vi "1WIRE_ROM_SEARCH.vi"(7 "1-Wire DIO Pin":refnum<k21>="ConnectorA/DIO15", 8 "Error In":errorcluster) -> (0 "Error Out":errorcluster, 2 "ROM Array":u64[](array[numeric]))   [LabVIEW 2014]
uses:
  <vilib>/rvi/Emulation/niFpgaGetClockAttributes.vi
  <vilib>/rvi/Emulation/niFpgaSctlEmulationGetInTimedLoop.vi
  <vilib>/rvi/Emulation/niFpgaEmulationReportErrorSimple.vi
  <vilib>/rvi/Emulation/niFpgaCriticalErrorInLSC.vi
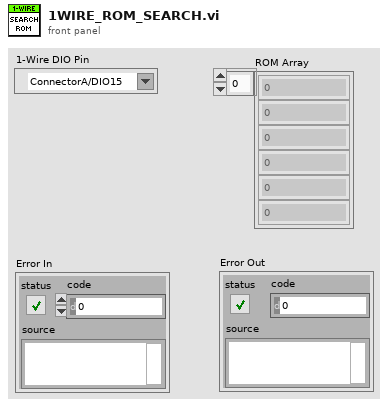
[diagram p1: front panel]
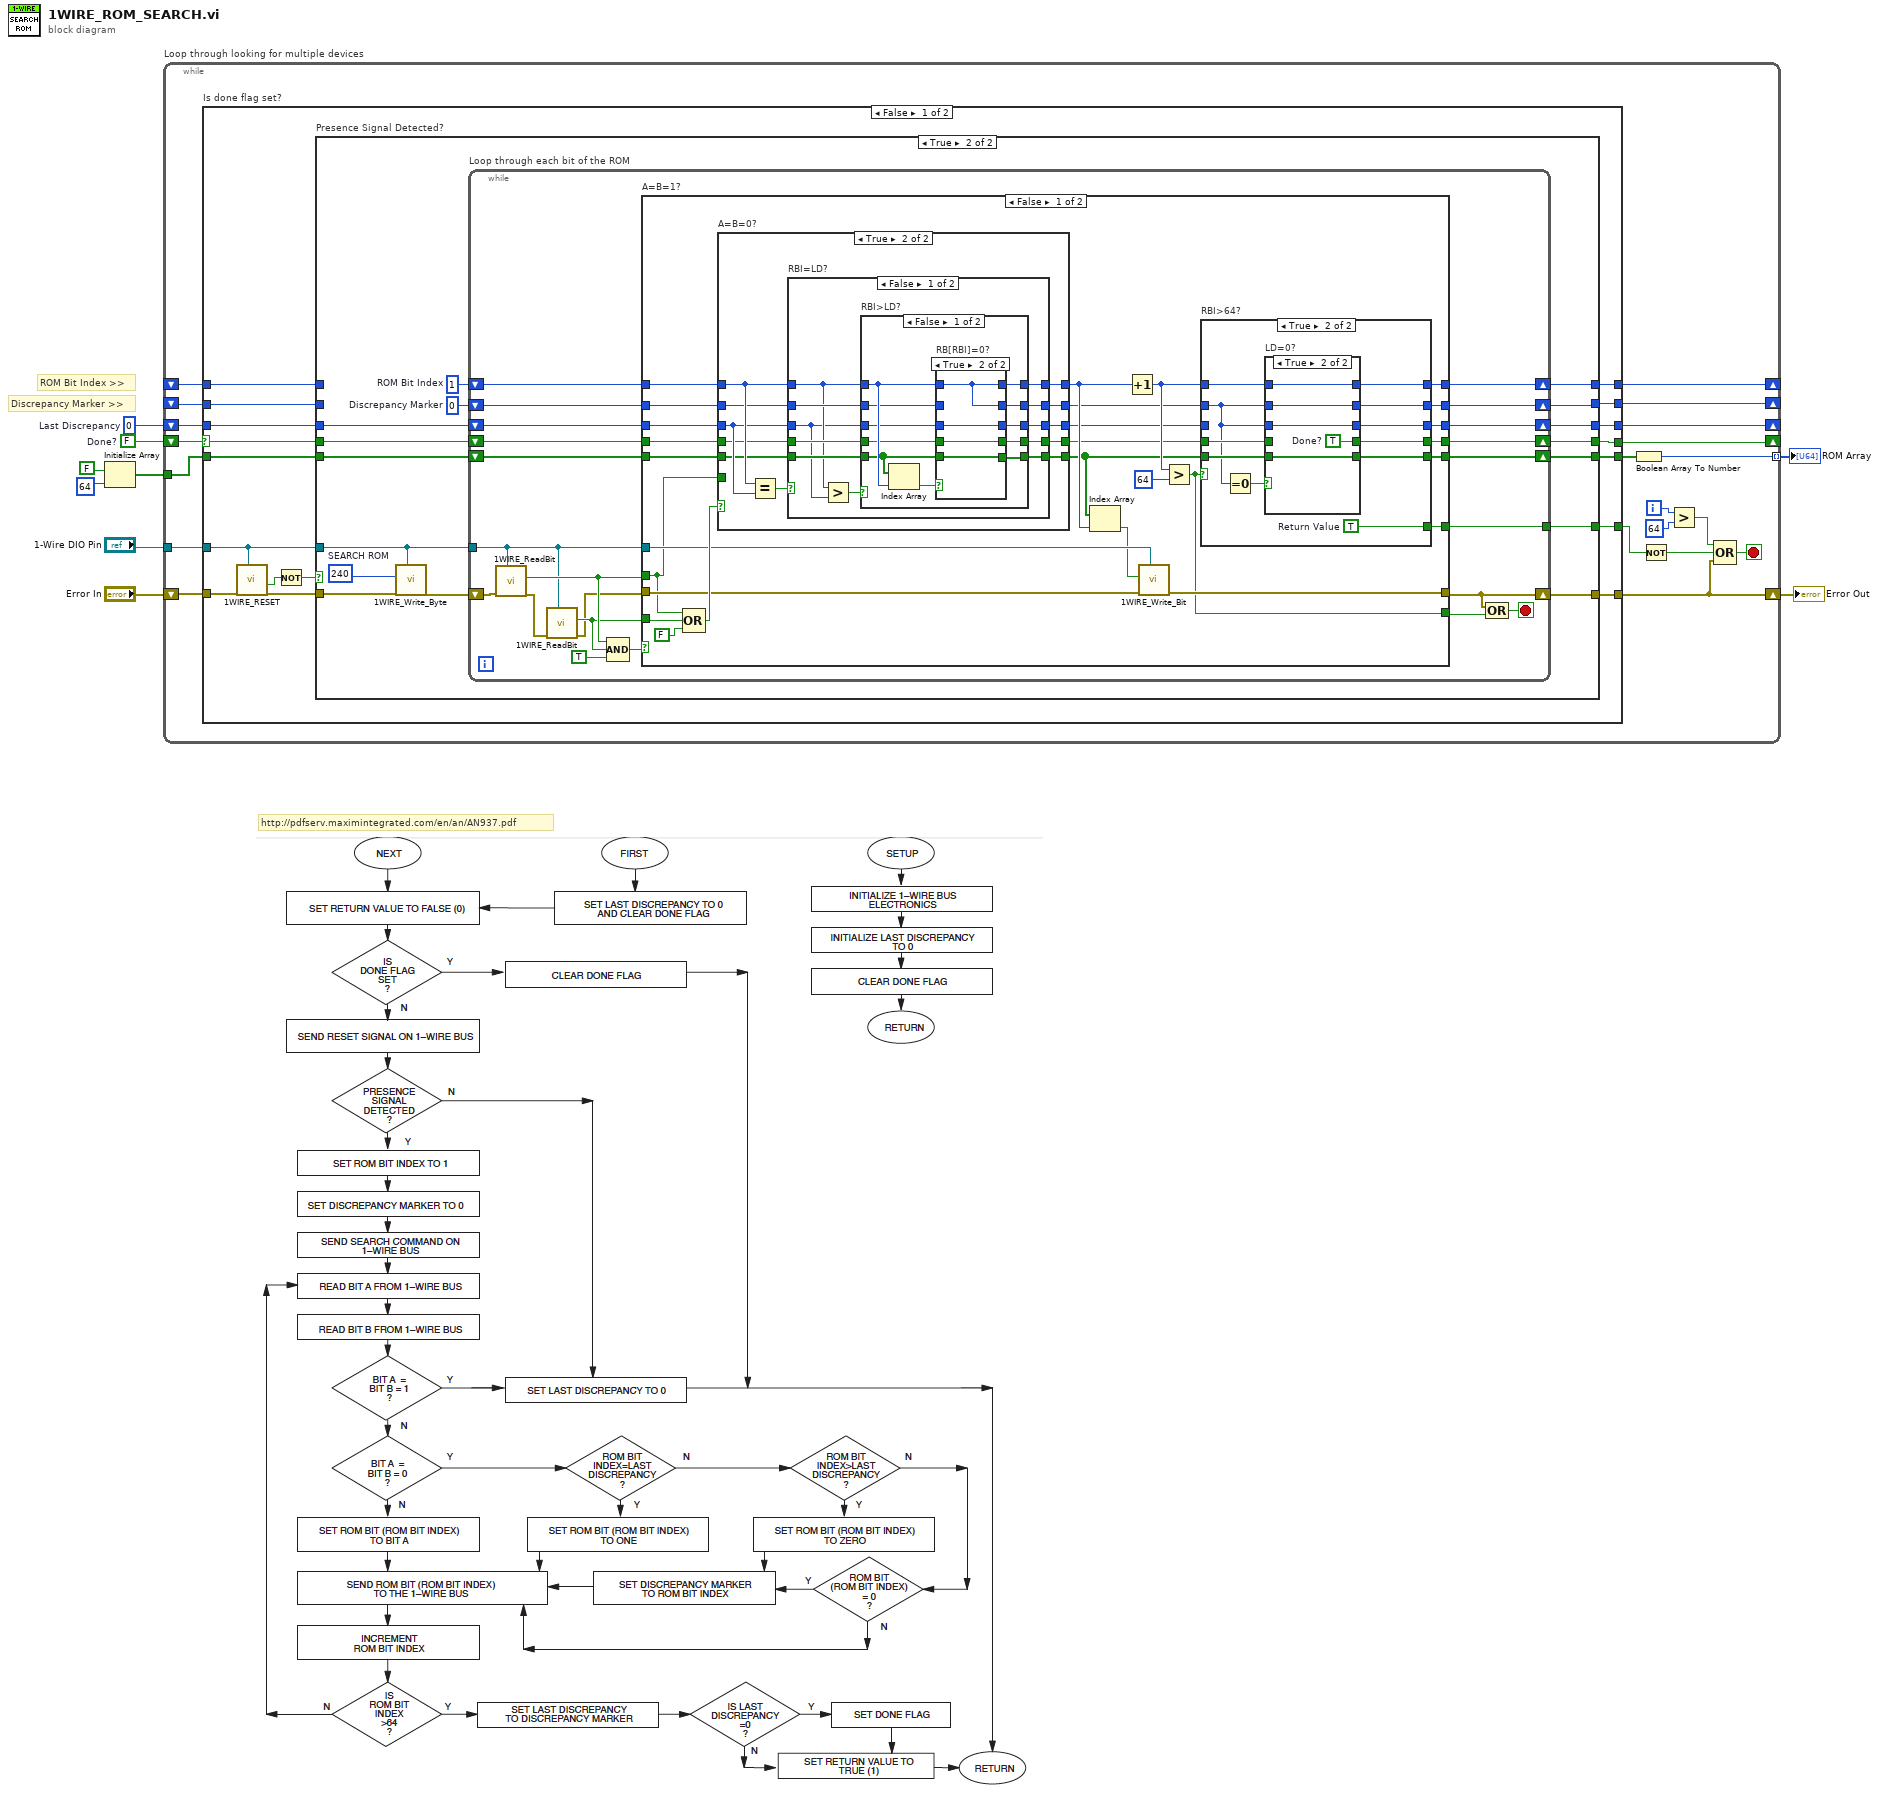
[diagram p0: block diagram]
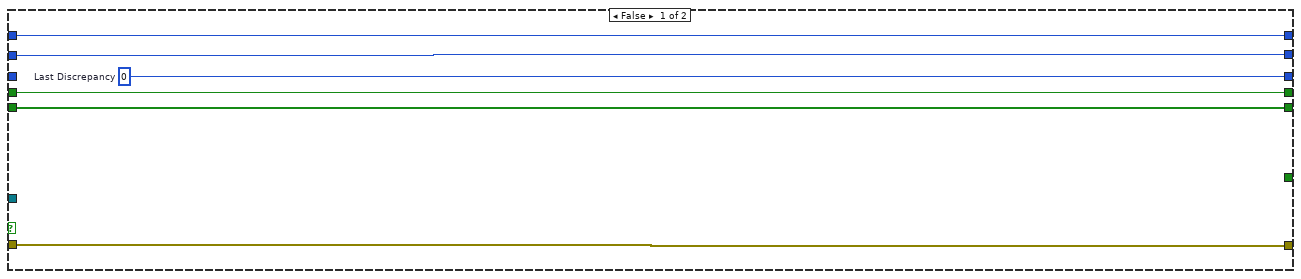
[diagram p2: hidden frame]
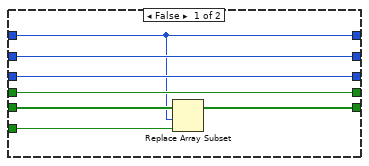
[diagram p5: hidden frame]
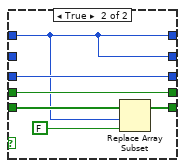
[diagram p7: hidden frame]
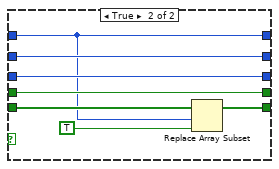
[diagram p8: hidden frame]
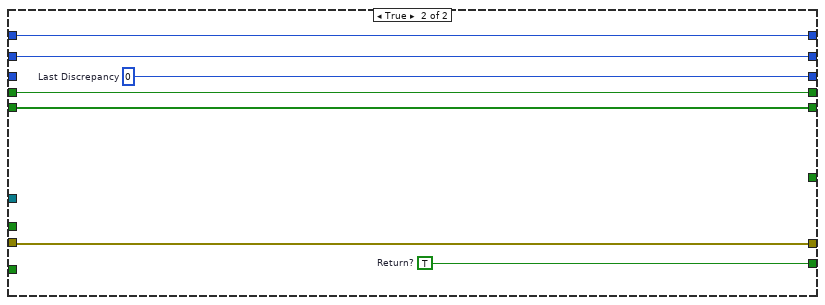
[diagram p9: hidden frame]
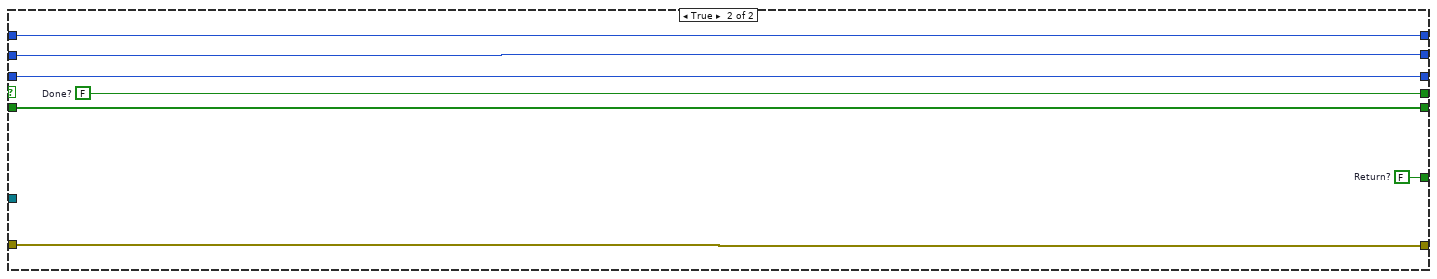
[diagram p10: hidden frame]
diagram:
  w6 = FALSE  # Done?
  w7 = i16 0  # Last Discrepancy
  # "http://pdfserv.maximintegrated.com/en/an/AN937.pdf"
  # "Discrepancy Marker >>"
  # "ROM Bit Index >>"
  n1 = Initialize Array(FALSE, 64 ("dimension size")) -> (w1:bool[])
  n2 = while "Loop through looking for multiple devices" {
    tunnel: [w25] -> w8 mode=indexing
    shift-right: [w23] -> _
    shift-left: w7 -> [w24]
    shift-right: [w21] -> _
    shift-left: w6 -> [w22]
    shift-right: [w20] -> _
    shift-left: _ -> [w18]
    shift-right: [w19] -> _
    shift-left: _ -> [w17]
    tunnel: "1-Wire DIO Pin" -> [w16]
    shift-right: [w27] -> w9
    shift-left: "Error In" -> [w15]
    tunnel: w1 -> [w14]
    i -> [w11]
    stop <- w13 stop-if-true
    n3 = case "Is done flag set?" shown="False" w22 {
      selector: w22 -> [w37 _]
      tunnel: [w36 w219] -> w21
      tunnel: w16 -> [w35 _]
      tunnel: [w42 w216] -> w27
      tunnel: w15 -> [w46 w216]
      tunnel: [w41 w217] -> w23
      tunnel: w18 -> [w40 w218]
      tunnel: [w39 w218] -> w20
      tunnel: w24 -> [w38 w217]
      tunnel: w17 -> [w34 w215]
      tunnel: [w33 w215] -> w19
      tunnel: w14 -> [w32 w214]
      tunnel: [w31 w214] -> w29
      tunnel: [w30 w213] -> w28
      frame False {
        n4 = call "1WIRE_RESET.vi"("1-Wire DIO Pin"=w35, "error in"=w46) -> ("error out"=w45:errorcluster, "0 = Device Present / 1=no"=w44:bool)  [unwired: 8 in]
        n5 = Not(x=w44) -> (.not. x?=w43:bool)
        n6 = case "Presence Signal Detected?" shown="True" w43 {
          tunnel: w45 -> [w52 w68]
          tunnel: [w52 w61] -> w42
          tunnel: [w51 w65] -> w41
          tunnel: w40 -> [w50 _]
          tunnel: [w50 w59] -> w39
          tunnel: w38 -> [_ w62]
          tunnel: w37 -> [w49 w64]
          tunnel: [w49 w63] -> w36
          tunnel: w35 -> [_ w54]
          tunnel: w34 -> [w48 _]
          tunnel: [w48 w57] -> w33
          tunnel: w32 -> [w47 w56]
          tunnel: [w47 w55] -> w31
          tunnel: [_ w53] -> w30
          frame False {
            w51 = i16 0  # Last Discrepancy
          }
          frame True {
            w58 = i16 0  # Discrepancy Marker
            w67 = u8 240  # SEARCH ROM
            w60 = i16 1  # ROM Bit Index
            n7 = call "1WIRE_Write_Byte.vi"("1-Wire DIO Pin"=w54, "error in"=w68, "Tx data"=w67) -> ("error out"=w66:errorcluster)  [unwired: 7 in, 1 out]
            n8 = while "Loop through each bit of the ROM" {
              tunnel: w54 -> [w73]
              shift-right: [w71] -> w61
              shift-left: w66 -> [w90]
              shift-right: [w84] -> w63
              shift-left: w64 -> [w85]
              shift-right: [w74] -> w55
              shift-left: w56 -> [w75]
              shift-right: [w78] -> w59
              shift-left: w60 -> [w79]
              shift-right: [w76] -> w57
              shift-left: w58 -> [w77]
              shift-right: [w86] -> w65
              shift-left: w62 -> [w83]
              tunnel: [w72] -> w53
              stop <- w69 stop-if-true
              n9 = call "1WIRE_ReadBit.vi"("1-Wire DIO Pin"=w73, "error in"=w90) -> ("error out"=w89:errorcluster, "Bit Read"=w82:bool)  [unwired: 8 in]
              n10 = call "1WIRE_ReadBit.vi"("1-Wire DIO Pin"=w73, "error in"=w89) -> ("error out"=w80:errorcluster, "Bit Read"=w81:bool)  [unwired: 8 in]
              n11 = Compound Arithmetic op=AND(w82, w81, TRUE ("value")) -> (w87:bool)
              n12 = case "A=B=1?" shown="False" w87 {
                tunnel: [w97 w212] -> w86
                tunnel: w85 -> [w114 w211]
                tunnel: [w95 w211] -> w84
                tunnel: [w92 w210] -> w70
                tunnel: w83 -> [w115 _]
                tunnel: w82 -> [w104 _]
                tunnel: w81 -> [w116 _]
                tunnel: w80 -> [w107 w209]
                tunnel: [w109 w209] -> w71
                tunnel: w79 -> [w112 w208]
                tunnel: [w101 w208] -> w78
                tunnel: w77 -> [w111 w207]
                tunnel: [w99 w207] -> w76
                tunnel: w75 -> [w110 w206]
                tunnel: [w93 w206] -> w74
                tunnel: w73 -> [w108 _]
                tunnel: [w91 _] -> w72
                frame False {
                  n13 = Compound Arithmetic op=OR(w104, w116, FALSE ("value")) -> (w113:bool)
                  n14 = case "A=B=0?" shown="True" w113 {
                    tunnel: w115 -> [w150 w156]
                    tunnel: [w150 w155] -> w98
                    tunnel: w114 -> [w149 w154]
                    tunnel: [w149 w153] -> w96
                    tunnel: w112 -> [w145 w160]
                    tunnel: [w145 w159] -> w106
                    tunnel: w111 -> [w148 w158]
                    tunnel: [w148 w157] -> w100
                    tunnel: w110 -> [w147 w152]
                    tunnel: [w146 w151] -> w94
                    tunnel: w104 -> [w144 _]
                    frame False {
                      n15 = Replace Array Subset(array=w147, new element=w144, index=w145) -> (w146:bool[])
                    }
                    frame True {
                      n16 = Equal?(x=w160, y=w156) -> (x = y?=w161:bool)
                      n17 = case "RBI=LD?" shown="False" w161 {
                        tunnel: w160 -> [w163 w200]
                        tunnel: [w172 w200] -> w159
                        tunnel: w158 -> [w171 w205]
                        tunnel: [w170 w205] -> w157
                        tunnel: w156 -> [w162 w204]
                        tunnel: [w169 w204] -> w155
                        tunnel: w154 -> [w168 w203]
                        tunnel: [w167 w203] -> w153
                        tunnel: w152 -> [w166 w202]
                        tunnel: [w165 w201] -> w151
                        frame False {
                          n18 = Greater?(x=w163, y=w162) -> (0:w164:bool)
                          n19 = case "RBI>LD?" shown="False" w164 {
                            tunnel: [w181 w193] -> w172
                            tunnel: w163 -> [w182 w193]
                            tunnel: w171 -> [w180 _]
                            tunnel: [w179 w193] -> w170
                            tunnel: w162 -> [w177 w198]
                            tunnel: [w178 w198] -> w169
                            tunnel: w168 -> [w176 w197]
                            tunnel: [w175 w197] -> w167
                            tunnel: w166 -> [w174 w196]
                            tunnel: [w173 w195] -> w165
                            frame False {
                              n20 = Index Array(array=w174, index=w182) -> (element=w183:bool)
                              n21 = case "RB[RBI]=0?" shown="True" w183 {
                                tunnel: w182 -> [w188 w189]
                                tunnel: [w188 w189] -> w181
                                tunnel: w180 -> [w187 _]
                                tunnel: [w187 w189] -> w179
                                tunnel: [w186 w192] -> w178
                                tunnel: w177 -> [w186 w192]
                                tunnel: w176 -> [w185 w191]
                                tunnel: [w185 w191] -> w175
                                tunnel: [w184 w190] -> w173
                                tunnel: w174 -> [w184 w190]
                                frame False {
                                }
                                frame True {
                                }
                              }
                            }
                            frame True {
                              n22 = Replace Array Subset(array=w196, new element=FALSE ("new element/subarray"), index=w193) -> (w195:bool[])
                            }
                          }
                        }
                        frame True {
                          n23 = Replace Array Subset(array=w202, new element=TRUE ("new element/subarray"), index=w200) -> (w201:bool[])
                        }
                      }
                    }
                  }
                  n24 = Index Array(array=w94, index=w106) -> (element=w105:bool)
                  n25 = Increment(x=w106) -> (x+1=w102:i16)
                  n26 = call "1WIRE_Write_Bit.vi"("1-Wire DIO Pin"=w108, "Error In"=w107, "Bit"=w105) -> ("Error Out"=w109:errorcluster)  [unwired: 8 in]
                  n27 = Greater?(x=w102, y=i16 64) -> (0:w92:bool)
                  n28 = case "RBI>64?" shown="True" w92 {
                    tunnel: w102 -> [w122 w131]
                    tunnel: [w122 w130] -> w101
                    tunnel: w100 -> [w121 w125]
                    tunnel: [w121 w132] -> w99
                    tunnel: w98 -> [w120 _]
                    tunnel: [w120 w133] -> w97
                    tunnel: w96 -> [w119 w129]
                    tunnel: [w119 w128] -> w95
                    tunnel: w94 -> [w118 w127]
                    tunnel: [w118 w126] -> w93
                    tunnel: [_ w123] -> w91
                    frame False {
                    }
                    frame True {
                      w123 = TRUE  # Return Value
                      n29 = Equal To 0?(x=w125) -> (x = 0?=w124:bool)
                      n30 = case "LD=0?" shown="True" w124 {
                        tunnel: [w134 w140] -> w133
                        tunnel: w125 -> [w136 w143]
                        tunnel: [w136 w143] -> w132
                        tunnel: w131 -> [w135 w142]
                        tunnel: [w135 w142] -> w130
                        tunnel: w129 -> [w137 _]
                        tunnel: [w137 w139] -> w128
                        tunnel: w127 -> [w138 w141]
                        tunnel: [w138 w141] -> w126
                        tunnel: w125 -> [w134 w140]
                        frame False {
                        }
                        frame True {
                          w139 = TRUE  # Done?
                        }
                      }
                    }
                  }
                }
                frame True {
                  w210 = TRUE  # Return?
                  w212 = i16 0  # Last Discrepancy
                }
              }
              n31 = Compound Arithmetic op=OR(w71, w70) -> (w69:bool)
            }
          }
        }
      }
      frame True {
        w213 = FALSE  # Return?
        w219 = FALSE  # Done?
      }
    }
    n32 = Boolean Array To Number(Boolean array=w29) -> (number=w25:u64)
    n33 = Not(x=w28) -> (.not. x?=w26:bool)
    n34 = Greater?(x=w11, y=64) -> (0:w12:bool)
    n35 = Compound Arithmetic op=OR(w12, w26, w27) -> (w13:bool)
  }
  "Error Out" <- w9
  "ROM Array" <- w8
